vi "setUp.vi"(8 "error in (no error)":errorcluster, 11 "reference in":refnum<class "Test Network Stream Disconnect.lvclass">) -> (0 "error out":errorcluster, 3 "reference out":refnum<class "Test Network Stream Disconnect.lvclass">)   [LabVIEW 2020, in "Test Network Stream Disconnect.lvclass"]
doc: "setUp runs prior to the test method during test execution. Use this method to initialize any object data required by your tests."
uses:
  Test Network Stream Disconnect.lvclass
  <vilib>/addons/_JKI Toolkits/VI Tester/TestCase.llb/TestCase.lvclass
  Source/Protocols/Network Stream Strategy/Network Stream Initiator/Network Stream Initiator.lvclass
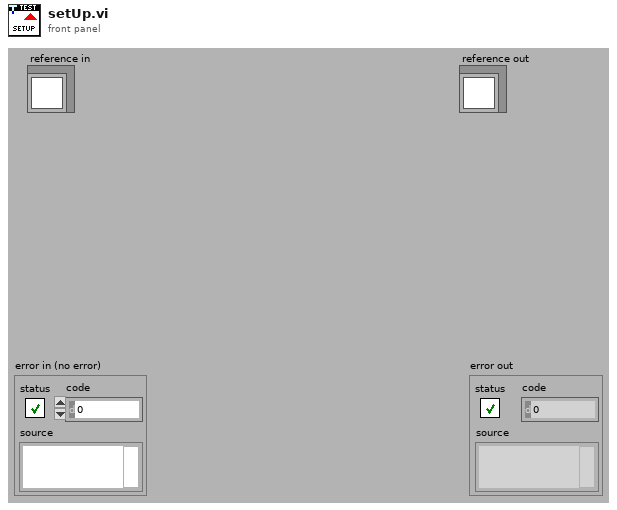
[diagram p1: front panel]
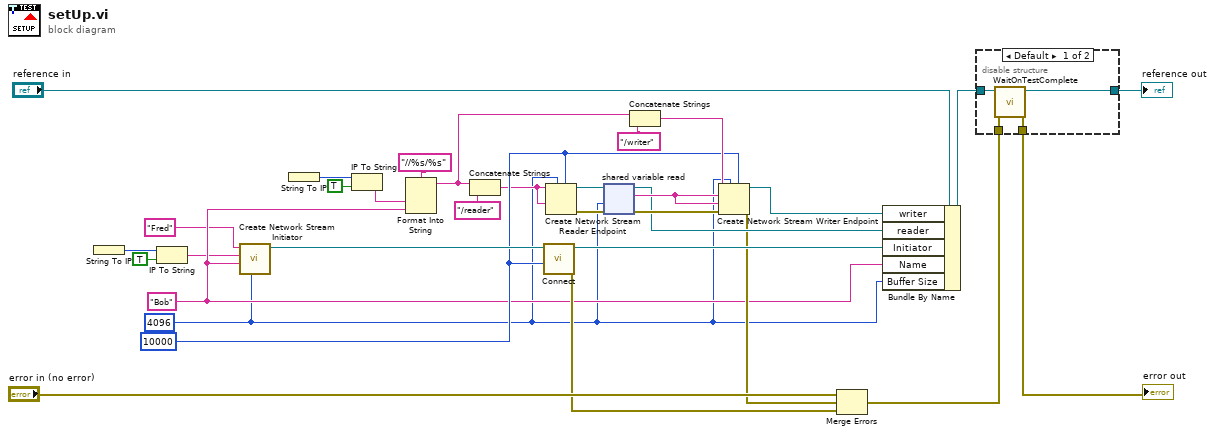
[diagram p0: block diagram]
diagram:
  w17 = 10000 ("timeout")
  w1 = 4096 ("Buffer Size")
  w4 = "Bob" ("Remote Name")
  n1 = String To IP() -> (0:w27:u32)  [unwired: 1 in]
  n2 = IP To String(1:TRUE ("dot notation? (F)"), 2:w27) -> (0:w3:string)
  n3 = call "Create Network Stream Initiator.vi"("Buffer Size"=w1, "Remote Name"=w4, "Remote Address"=w3, "Name"="Fred") -> ("Network Stream Initiator out"=w25:refnum<class "Network Stream Initiator.lvclass">)  [unwired: 7 in]
  n4 = String To IP() -> (0:w12:u32)  [unwired: 1 in]
  n5 = IP To String(1:TRUE ("dot notation? (F)"), 2:w12) -> (0:w14:string)
  n6 = Format Into String(format string="//%s/%s", w14, w4) -> (resulting string=w23:string)  [unwired: 2 in, 1 out]
  n7 = Concatenate Strings(w23, "/reader" ("format string")) -> (w15:string)
  n8 = call-dynamic "Connect.vi"("timeout"=w17, "Network Stream Initiator in"=w25) -> ("error out"=w6:errorcluster, "Network Stream Initiator out"=w10:refnum<class "Network Stream Initiator.lvclass">)  [unwired: 8 in]
  n9 = Create Network Stream Reader Endpoint(5:w17, 7:w1, 9:w15, 11:w15) -> (0:w18:errorcluster, 3:w19:refnum<k21>)  [unwired: 3 in]
  n10 = shared-variable-read(w19, w18, w1) -> (w9:refnum<k21>, w20:errorcluster, w21:string)  [unwired: 1 out]
  n11 = Concatenate Strings(w23, "/writer" ("format string")) -> (w24:string)
  n12 = Create Network Stream Writer Endpoint(5:w17, 7:w1, 8:w20, 9:w21, 10:w21, 11:w24) -> (0:w5:errorcluster, 3:w8:refnum<k21>)  [unwired: 1 in]
  n13 = Merge Errors("error in (no error)", w5, w6) -> (w7:errorcluster)
  n14 = Bundle By Name(cluster="reference in", "writer"=w8, "reader"=w9, "Initiator"=w10, "Name"=w4, "Buffer Size"=w1) -> (w28:refnum<class "Test Network Stream Disconnect.lvclass">)
  n15 = disable-structure shown="Default" {
    disable-tunnel: w7 -> [w36 w37]
    disable-tunnel: [w35 w37] -> w31
    disable-tunnel: [w34 w38] -> w29
    disable-tunnel: w28 -> [w33 w38]
    frame condition #0 (active) {
      n16 = call <vilib>:"WaitOnTestComplete.vi"("error in (no error)"=w36, "TestCase in"=w33) -> ("error out"=w35:errorcluster, "TestCase out"=w34:refnum<class "Test Network Stream Disconnect.lvclass">)  [unwired: 8 in]
    }
    frame condition #1 {
    }
  }
  "error out" <- w31
  "reference out" <- w29
